vi "Anritsu_MT8852B_YYLL_TesingINS.vi"(8 "error in":errorcluster, 9 "Test Timeout":dbl, 11 "VISA resource in":refnum<visa-resource-name>) -> (0 "error out":errorcluster, 1 "TestStopString":string, 2 "test done to read":bool, 3 "VISA resource out":refnum<visa-resource-name>)   [LabVIEW 2017]
uses:
  18eb8796-3083-4835-82b5-6d92ff9e593b.vi
panel:
  out "times":dbl
  out "ins type":T1
  out "Show":bool
  out "*INS?":u8 format="%.0b"
  # "TESTING>>>\n*INS?"
  # "MT8852B"
  # "Anritsu"
  # "YYLL"
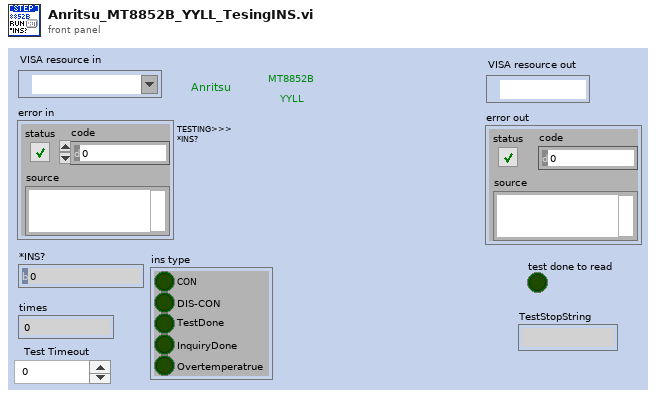
[diagram p1: front panel]
types:
  T1 = cluster{"CON":bool, "DIS-CON":bool, "TestDone":bool, "InquiryDone":bool, "Overtemperatrue":bool}
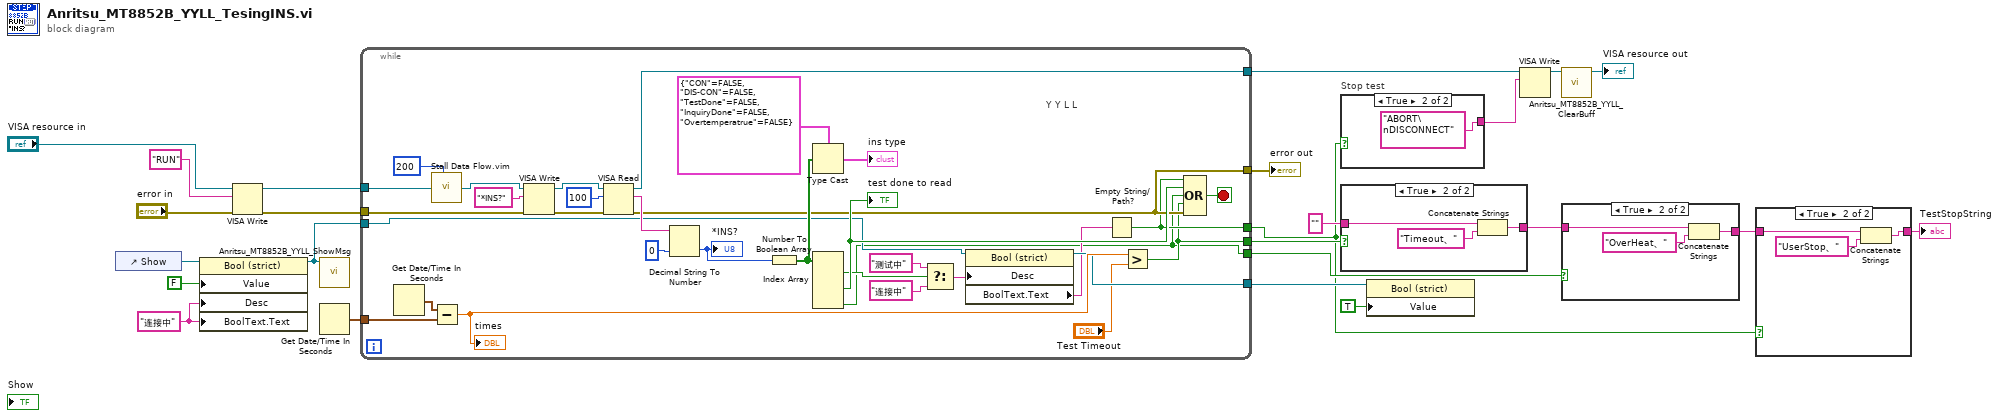
[diagram p0: block diagram]
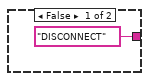
[diagram p5: hidden frame]
diagram:
  w12 = "连接中" ("String")
  n1 = control-ref of="Show"() -> (w17:refnum<vi>)
  n2 = property on="Property Node" class="Bool (strict)"(reference=w17, "Value"=FALSE, "Desc"=w12, "BoolText.Text"=w12) -> (reference out=w15:refnum<vi>)  [unwired: 1 in, 1 out]
  n3 = VISA Write(VISA resource name="VISA resource in", write buffer="RUN" ("write buffer (\"\")"), error in (no error)="error in") -> (VISA resource name out=w22:refnum<visa-resource-name>, error out=w21:errorcluster)  [unwired: 1 out]
  n4 = call "Anritsu_MT8852B_YYLL_ShowMsg.vi"("reference out"=w15) -> ()  [unwired: 11 in]
  n5 = Get Date/Time In Seconds() -> (seconds since 1Jan1904=w23:timestamp)
  n6 = while {
    tunnel: w22 -> [w47]
    tunnel: [w45] -> w11
    tunnel: w21 -> [w46]
    tunnel: w23 -> [w54]
    tunnel: [w30] -> w18
    tunnel: w15 -> [w35]
    tunnel: [w36] -> w14
    tunnel: [w28] -> w2
    tunnel: [w27] -> w7
    tunnel: [w26] -> w4
    stop <- w56 stop-if-true
    # "Y Y L L"
    n7 = Get Date/Time In Seconds() -> (seconds since 1Jan1904=w55:timestamp)
    n8 = call "Stall Data Flow.vim"("value in"=w47, "milliseconds to wait"=u32 200) -> ("value out"=w44:refnum<visa-resource-name>)  [unwired: 1 out]
    n9 = Subtract(x=w55, y=w54) -> (x-y=w53:dbl)
    "times" <- w53
    n10 = VISA Write(VISA resource name=w44, write buffer="*INS?" ("write buffer (\"\")"), error in (no error)=w46) -> (VISA resource name out=w49:refnum<visa-resource-name>, error out=w50:errorcluster)  [unwired: 1 out]
    n11 = VISA Read(VISA resource name=w49, byte count=u32 100 ("byte count (0)"), error in (no error)=w50) -> (VISA resource name out=w45:refnum<visa-resource-name>, read buffer=w52:string, error out=w30:errorcluster)  [unwired: 1 out]
    n12 = Decimal String To Number(string=w52, default (0L)=u8 0 ("default (0 I32)")) -> (number=w41:u8)  [unwired: 1 in, 1 out]
    "*INS?" <- w41
    n13 = Number To Boolean Array(number=w41) -> (Boolean array=w38:bool[])
    n14 = Type Cast(type=T1 {"CON"=FALSE, "DIS-CON"=FALSE, "TestDone"=FALSE, "InquiryDone"=FALSE, "Overtemperatrue"=FALSE}, x=w38) -> (*(type *) &x=→"ins type":T1)
    n15 = Index Array(array=w38) -> (element #1=w34:bool, element #3=w40:bool, element #5=w26:bool)  [unwired: 5 in, 2 out]
    "test done to read" <- w40
    n16 = Select(t="测试中", s=w34, f="连接中") -> (s? t:f=w32:string)
    n17 = property on="Property Node" class="Bool (strict)"(reference=w35, "Desc"=w32) -> (reference out=w36:refnum<vi>, "BoolText.Text"=w29:string)  [unwired: 1 in, 1 out]
    n18 = Empty String/Path?(string/path=w29) -> (empty?=w28:bool)
    n19 = Greater?(x=w53, y="Test Timeout") -> (0:w27:bool)
    n20 = Compound Arithmetic op=OR(w28, w40, w26, w27, w30) -> (w56:bool)
  }
  "error out" <- w18
  n21 = case "Stop test" shown="True" w2 {
    tunnel: ["DISCONNECT" ("write buffer (\"\")") "ABORT\nDISCONNECT" ("write buffer (\"\")")] -> w9
    frame False {
    }
    frame True {
    }
  }
  n22 = case shown="True" w7 {
    tunnel: "" -> [w59 w62]
    tunnel: [w59 w60] -> w5
    frame False {
    }
    frame True {
      n23 = Concatenate Strings(w62, "Timeout、" ("string")) -> (w60:string)
    }
  }
  n24 = property on="Property Node" class="Bool (strict)"(reference=w14, "Value"=TRUE) -> ()  [unwired: 1 in, 2 out]
  n25 = VISA Write(VISA resource name=w11, write buffer=w9) -> (VISA resource name out=w8:refnum<visa-resource-name>)  [unwired: 1 in, 2 out]
  n26 = call "Anritsu_MT8852B_YYLL_ClearBuff.vi"("VISA resource name"=w8) -> ("VISA resource name 2"=→"VISA resource out":refnum<visa-resource-name>)  [unwired: 8 in, 2 out]
  n27 = case shown="True" w4 {
    tunnel: w5 -> [w63 w66]
    tunnel: [w63 w64] -> w3
    frame False {
    }
    frame True {
      n28 = Concatenate Strings(w66, "OverHeat、" ("string")) -> (w64:string)
    }
  }
  n29 = case shown="True" w2 {
    tunnel: w3 -> [w67 w70]
    tunnel: [w67 w68] -> w1
    frame False {
    }
    frame True {
      n30 = Concatenate Strings(w70, "UserStop、" ("string")) -> (w68:string)
    }
  }
  "TestStopString" <- w1
